vi "INA219 Init & Config.vi"(7 "I2C Channel":u8, 8 "error in (no error)":errorcluster, 9 "INA219 Config Options":T1={"I2C"={"Slave Address"=64, "Channel"=0}, "Reset bit"=0, "Bus Voltage Range"=1, "PGA/Shunt Voltage Gain"=3, "Bus Voltage ADC Settings"=8, "Shunt Voltage ADC Settings"=3, "Mode"=7, "Calibration Value"=4096, "Online"=FALSE, "Shunt Resistor"=0.1} {"Shunt Resistor" format="%#_g ohm"; "I2C"."Slave Address" format="%.0x"; "Calibration Value" format="%.0x"; "Mode" items=["Power Down", "Shunt Voltage, Triggered", "Bus Voltage, Triggered", "Shunt & Bus, Triggered", "ADC Off (Disabled)", "Shunt Voltage, Continuous", "Bus Voltage, Continuous", "Shunt & Bus Voltage, Continuous"]; "Shunt Voltage ADC Settings" items=["9-bit, 84us conversion time"=0, "10-bit, 148us conversion time"=1, "11-bit, 276us conversion time"=2, "12-bit, 532us conversion time"=3, "1x12-bit, 532us conversion time"=8, "2x12-bit averaged, 1.06ms conversion time"=9, "4x12-bit averaged, 2.13ms conversion time"=10, "8x12-bit averaged, 4.26ms conversion time"=11, "16x12-bit averaged, 8.51ms conversion time"=12, "32x12-bit averaged, 17.02ms conversion time"=13, "64x12-bit averaged, 34.05ms conversion time"=14, "128x12-bit averaged, 68.10ms conversion time"=15]; "Bus Voltage ADC Settings" items=["9-bit, 84us conversion time"=0, "10-bit, 148us conversion time"=1, "11-bit, 276us conversion time"=2, "12-bit, 532us conversion time"=3, "1x12-bit, 532us conversion time"=8, "2x12-bit averaged, 1.06ms conversion time"=9, "4x12-bit averaged, 2.13ms conversion time"=10, "8x12-bit averaged, 4.26ms conversion time"=11, "16x12-bit averaged, 8.51ms conversion time"=12, "32x12-bit averaged, 17.02ms conversion time"=13, "64x12-bit averaged, 34.05ms conversion time"=14, "128x12-bit averaged, 68.10ms conversion time"=15]; "PGA/Shunt Voltage Gain" items=["Gain 1, +/-40mV", "Gain 2, +/-80mV", "Gain 3, +/-160mV", "Gain 4, +/-320mV"]; "Bus Voltage Range" items=["0-16V Range", "0-32V Range"]; "Reset bit" items=["Do Not Reset", "Reset"]}, 10 "I2C Slave Address":u8=64 format="%.0x", 11 "LINX Resource in":T2) -> (0 "error out":errorcluster, 1 "INA219 Config Options":T1={"I2C"={"Slave Address"=64, "Channel"=0}, "Reset bit"=0, "Bus Voltage Range"=0, "PGA/Shunt Voltage Gain"=0, "Bus Voltage ADC Settings"=0, "Shunt Voltage ADC Settings"=0, "Mode"=0, "Calibration Value"=4096, "Online"=FALSE, "Shunt Resistor"=0.1} {"Shunt Resistor" format="%#_g ohm"; "I2C"."Slave Address" format="%.0x"; "Calibration Value" format="%.0x"; "Mode" items=["Power Down", "Shunt Voltage, Triggered", "Bus Voltage, Triggered", "Shunt & Bus, Triggered", "ADC Off (Disabled)", "Shunt Voltage, Continuous", "Bus Voltage, Continuous", "Shunt & Bus Voltage, Continuous"]; "Shunt Voltage ADC Settings" items=["9-bit, 84us conversion time"=0, "10-bit, 148us conversion time"=1, "11-bit, 276us conversion time"=2, "12-bit, 532us conversion time"=3, "1x12-bit, 532us conversion time"=8, "2x12-bit averaged, 1.06ms conversion time"=9, "4x12-bit averaged, 2.13ms conversion time"=10, "8x12-bit averaged, 4.26ms conversion time"=11, "16x12-bit averaged, 8.51ms conversion time"=12, "32x12-bit averaged, 17.02ms conversion time"=13, "64x12-bit averaged, 34.05ms conversion time"=14, "128x12-bit averaged, 68.10ms conversion time"=15]; "Bus Voltage ADC Settings" items=["9-bit, 84us conversion time"=0, "10-bit, 148us conversion time"=1, "11-bit, 276us conversion time"=2, "12-bit, 532us conversion time"=3, "1x12-bit, 532us conversion time"=8, "2x12-bit averaged, 1.06ms conversion time"=9, "4x12-bit averaged, 2.13ms conversion time"=10, "8x12-bit averaged, 4.26ms conversion time"=11, "16x12-bit averaged, 8.51ms conversion time"=12, "32x12-bit averaged, 17.02ms conversion time"=13, "64x12-bit averaged, 34.05ms conversion time"=14, "128x12-bit averaged, 68.10ms conversion time"=15]; "PGA/Shunt Voltage Gain" items=["Gain 1, +/-40mV", "Gain 2, +/-80mV", "Gain 3, +/-160mV", "Gain 4, +/-320mV"]; "Bus Voltage Range" items=["0-16V Range", "0-32V Range"]; "Reset bit" items=["Do Not Reset", "Reset"]}, 3 "LINX Resource out":T2)   [LabVIEW 2018]
uses:
  <vilib>/MakerHub/LINX/Private/Type Defs/Platform.ctl
  <vilib>/MakerHub/LINX/Private/Type Defs/Interface.ctl
  <vilib>/MakerHub/LINX/Private/Device/Type Defs/TCP Config.ctl
  <vilib>/MakerHub/LINX/Private/Device/Type Defs/Channels.ctl
  <vilib>/MakerHub/LINX/Private/Device/Type Defs/LINX Device Config.ctl
  <vilib>/MakerHub/LINX/Private/Type Defs/LINX Ref.ctl
  INA219 Config Options.ctl
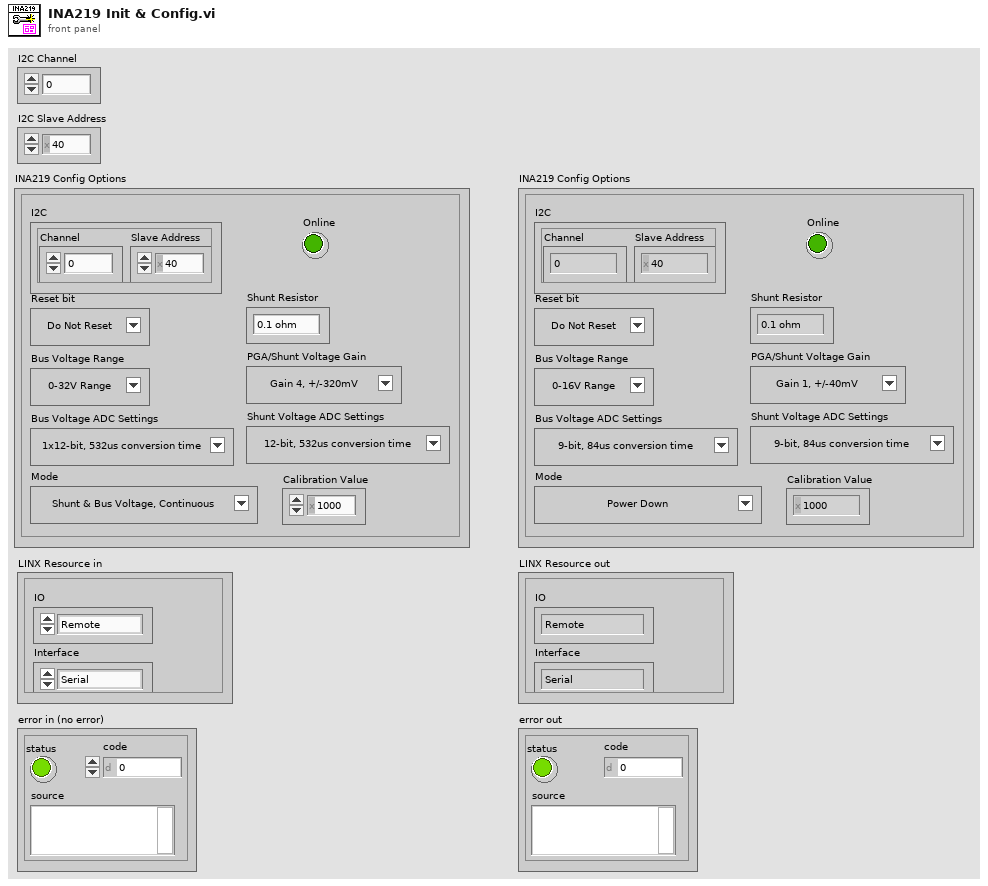
[diagram p1: front panel]
types:
  T1 = typedef "INA219 Config Options.ctl" = cluster{"I2C":cluster{"Slave Address":u8, "Channel":u8}, "Reset bit":u8, "Bus Voltage Range":u8, "PGA/Shunt Voltage Gain":u8, "Bus Voltage ADC Settings":u8, "Shunt Voltage ADC Settings":u8, "Mode":u8, "Calibration Value":u16, "Online":bool, "Shunt Resistor":dbl}
  T2 = typedef "LMH-LINX.lvlib/LINX Ref.ctl" = cluster{"IO":T3, "Interface":T4, "LINX Device Config":T5}
  T3 = typedef "LMH-LINX.lvlib/Platform.ctl" = enum16{"Remote", "Local"}
  T4 = typedef "LMH-LINX.lvlib/Interface.ctl" = enum16{"Serial", "TCP"}
  T5 = typedef "LMH-LINX.lvlib/Device.lvlib/LINX Device Config.ctl" = cluster{"Interface":T4, "COM Port":refnum<visa-resource-name>, "TCP Configuration":T6, "Device Family":u8, "Device ID":u8, "Device Name":string, "TCP Ref":refnum<k5>, "Channels":T7}
  T6 = typedef "LMH-LINX.lvlib/Device.lvlib/TCP Config.ctl" = cluster{"IP Address":string, "Port":u16}
  T7 = typedef "LMH-LINX.lvlib/Channels.ctl" = cluster{"DI":u8[], "DO":u8[], "AI":u8[], "AO":u8[], "PWM":u8[], "QE":u8[], "UART":u8[], "I2C 2":u8[], "SPI":u8[], "CAN":u8[], "Servo":u8[], "AI Ref (V)":dbl, "AI Resolution (Bits)":u8, "AO Ref (V)":dbl, "AO Resolution (Bits)":u8}
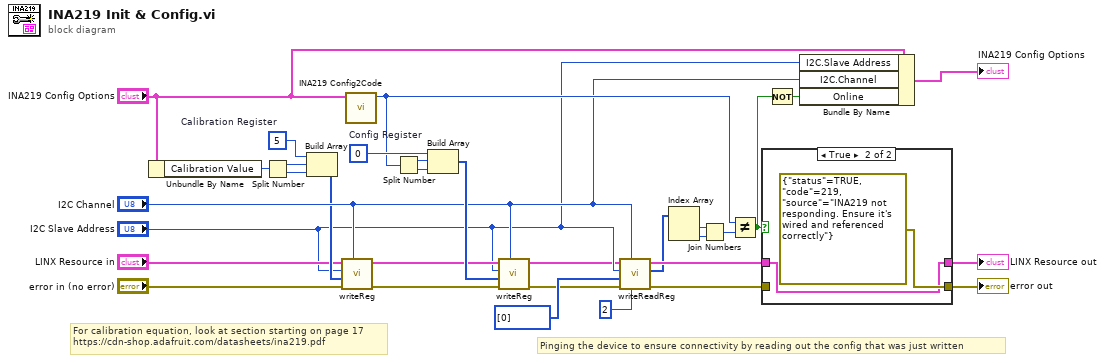
[diagram p0: block diagram]
diagram:
  w30 = u8 5  # Calibration Register
  w32 = u8 0  # Config Register
  # "Pinging the device to ensure connectivity by reading out the config that was just written"
  # "For calibration equation, look at section starting on page 17\nhttps://cdn-shop.adafruit.com/datasheets/ina219.pdf"
  n1 = Unbundle By Name("INA219 Config Options") -> ("Calibration Value"=w22:u16)
  n2 = Split Number(x=w22) -> (hi(x)=w27:u8, lo(x)=w26:u8)
  n3 = Build Array(w30, w27, w26) -> (w9:u8[])
  n4 = call "writeReg.vi"("I2C Channel"="I2C Channel", "error in"="error in (no error)", "Data"=w9, "I2C Slave Address"="I2C Slave Address", "LINX Resource in"="LINX Resource in") -> ("error out"=w23:errorcluster, "LINX Resource"=w24:T2)  [unwired: 5 in]
  n5 = call "INA219 Config2Code.vi"("INA219 Config Options"="INA219 Config Options") -> ("Config Code"=w20:u16)  [unwired: 10 in]
  n6 = Split Number(x=w20) -> (hi(x)=w28:u8, lo(x)=w29:u8)
  n7 = Build Array(w32, w28, w29) -> (w31:u8[])
  n8 = call "writeReg.vi"("I2C Channel"="I2C Channel", "error in"=w23, "Data"=w31, "I2C Slave Address"="I2C Slave Address", "LINX Resource in"=w24) -> ("error out"=w5:errorcluster, "LINX Resource"=w4:T2)  [unwired: 5 in]
  n9 = call "writeReadReg.vi"("Bytes To Read"=u8 2, "I2C Channel"="I2C Channel", "error in"=w5, "Data"=u8[] [0], "I2C Slave Address"="I2C Slave Address", "LINX Resource in"=w4) -> ("error out"=w19:errorcluster, "Bytes Read"=w13:u8[], "LINX Resource out"=w14:T2)  [unwired: 3 in]
  n10 = Index Array(array=w13) -> (element #1=w11:u8, element #2=w10:u8)  [unwired: 2 in]
  n11 = Join Numbers(hi=w11, lo=w10) -> ((hi.lo)=w21:u16)
  n12 = Not Equal?(x=w20, y=w21) -> (x != y?=w2:bool)
  n13 = case shown="True" w2 {
    tunnel: w19 -> [w34 _]
    tunnel: [w34 errorcluster {"status"=TRUE, "code"=219, "source"="INA219 not responding. Ensure it's wired and referenced correctly"} ("error constant")] -> w18
    tunnel: [w33 w35] -> w15
    tunnel: w14 -> [w33 w35]
    frame False {
    }
    frame True {
    }
  }
  "error out" <- w18
  "LINX Resource out" <- w15
  n14 = Not(x=w2) -> (.not. x?=w1:bool)
  n15 = Bundle By Name(cluster="INA219 Config Options", "I2C.Slave Address"="I2C Slave Address", "I2C.Channel"="I2C Channel", "Online"=w1) -> (→"INA219 Config Options":T1)
